vi "Tosca-Set Next Adapt Trial.vi"(0 "Track in":T4, 5 "change":bool, 7 "Track":T1, 9 "catch is tracked":bool) -> (4 "Track out":T4)   [LabVIEW 2020]
uses:
  Typedefs/Tosca-Adaptation Track State.ctl
  Typedefs/Tosca-Adaptation History Element.ctl
  Typedefs/Tosca-Adaptive Track.ctl
  Typedefs/Tosca-Simple Variable.ctl
  Tosca-Adapt Threshold Metric.ctl
  epl-vi-lib/Utility VIs/Array Manipulation VIs/Array-Dimensions (2D).vi
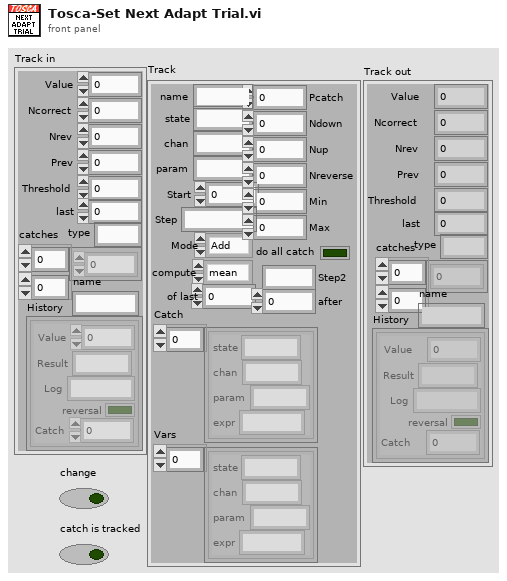
[diagram p1: front panel]
types:
  T1 = typedef "Tosca-Adaptive Track.ctl" = cluster{"state":string, "chan":string, "param":string, "Start":dbl, "Step":string, "Mode":enum16{"Add", "Multiply"}, "Pcatch":dbl, "Ndown":i32, "Nup":i32, "Nreverse":i32, "Min":dbl, "Max":dbl, "Catch":T2[], "do all catch":bool, "name":string, "Vars":T2[], "compute":T3, "of last":i32, "Step2":string, "after":i32}
  T2 = typedef "Tosca-Simple Variable.ctl" = cluster{"state":string, "chan":string, "param":string, "expr":string}
  T3 = typedef "Tosca-Adapt Threshold Metric.ctl" = enum16{"mean", "median"}
  T4 = typedef "Tosca-Adaptation Track State.ctl" = cluster{"Value":dbl, "Ncorrect":i32, "Nrev":i32, "Prev":dbl, "History":T5[], "Threshold":dbl, "last":i32, "type":string, "catches":dbl[][], "name":string}
  T5 = typedef "Tosca-Adaptation History Element.ctl" = cluster{"Value":dbl, "Result":string, "Log":string, "reversal":bool, "Catch":dbl}
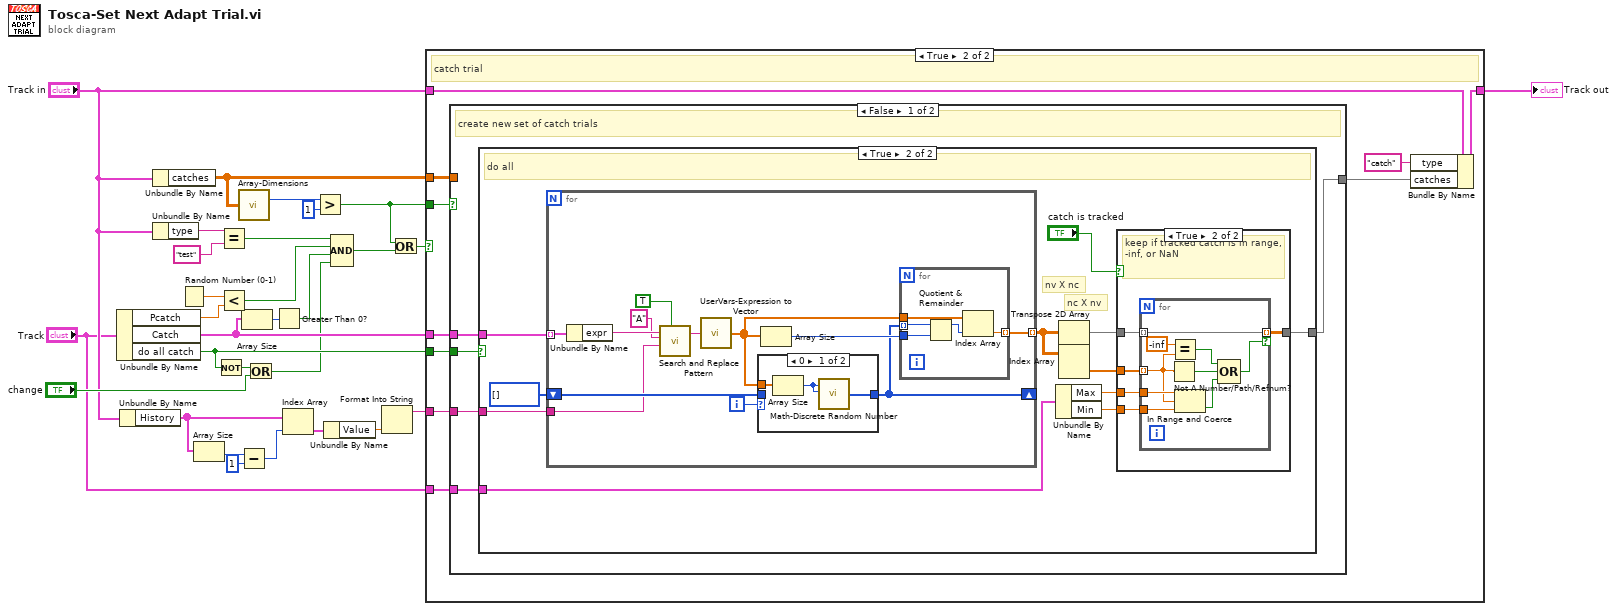
[diagram p0: block diagram]
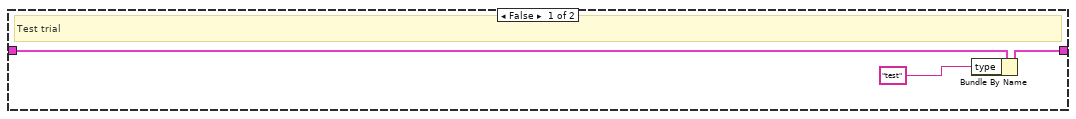
[diagram p2: hidden frame]
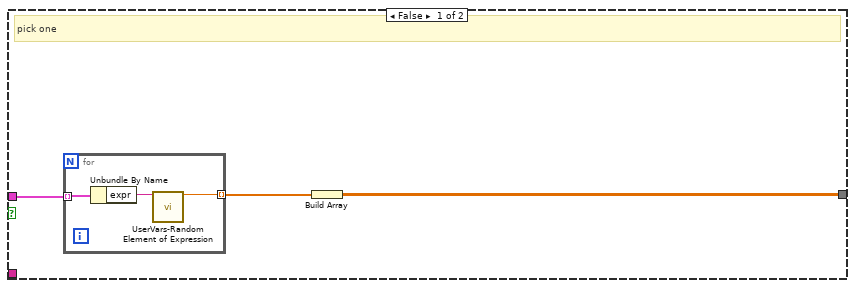
[diagram p3: hidden frame]
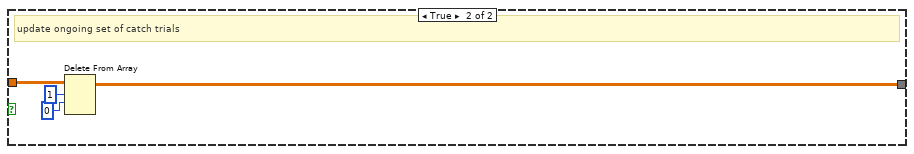
[diagram p6: hidden frame]
diagram:
  n1 = Unbundle By Name("Track") -> ("Pcatch"=w17:dbl, "Catch"=w16:T2[], "do all catch"=w13:bool)
  n2 = Unbundle By Name("Track in") -> ("History"=w4:T5[])
  n3 = Unbundle By Name("Track in") -> ("catches"=w21:dbl[][])
  n4 = Unbundle By Name("Track in") -> ("type"=w22:string)
  n5 = Random Number (0-1)() -> (number: 0 to 1=w24:dbl)
  n6 = Array Size(array=w4) -> (size(s)=w7:i32)
  n7 = Not(x=w13) -> (.not. x?=w12:bool)
  n8 = Equal?(x=w22, y="test") -> (x = y?=w25:bool)
  n9 = Less?(x=w24, y=w17) -> (x < y?=w26:bool)
  n10 = call-poly "Array-Dimensions.vi"("2D Array"=w21) -> ("# rows"=w19:i32)  [unwired: 13 in, 1 out]
  n11 = Subtract(x=w7, y=1) -> (x-y=w5:i32)
  n12 = Array Size(array=w16) -> (size(s)=w15:i32)
  n13 = Or(x=w12, y="change") -> (x .or. y?=w10:bool)
  n14 = Greater Than 0?(x=w15) -> (x > 0?=w14:bool)
  n15 = Index Array(array=w4, index=w5) -> (element=w3:T5)
  n16 = Greater?(x=w19, y=1) -> (0:w20:bool)
  n17 = Unbundle By Name(w3) -> ("Value"=w2:dbl)
  n18 = Compound Arithmetic op=AND(w25, w26, w14, w10) -> (w27:bool)
  n19 = Format Into String(w2) -> (resulting string=w8:string)  [unwired: 3 in, 1 out]
  n20 = Or(x=w20, y=w27) -> (x .or. y?=w28:bool)
  n21 = case shown="True" w28 {
    tunnel: "Track in" -> [w32 w42]
    tunnel: [w31 w39] -> w29
    tunnel: w21 -> [_ w40]
    tunnel: w20 -> [_ w41]
    tunnel: w16 -> [_ w36]
    tunnel: w13 -> [_ w35]
    tunnel: w8 -> [_ w34]
    tunnel: "Track" -> [_ w33]
    frame False {
      # "Test trial"
      n22 = Bundle By Name(cluster=w32, "type"="test") -> (w31:T4)
    }
    frame True {
      # "catch trial"
      n23 = case shown="False" w41 {
        tunnel: w40 -> [_ w104]
        tunnel: [w45 w102] -> w38
        tunnel: w36 -> [w46 _]
        tunnel: w35 -> [w47 _]
        tunnel: w34 -> [w44 _]
        tunnel: w33 -> [w43 _]
        frame False {
          # "create new set of catch trials"
          n24 = case shown="True" w47 {
            tunnel: w46 -> [w50 w64]
            tunnel: [w48 w56] -> w45
            tunnel: w44 -> [_ w63]
            tunnel: w43 -> [_ w62]
            frame False {
              # "pick one"
              n25 = for {
                tunnel: w50 -> [w53] mode=indexing
                tunnel: [w51] -> w49 mode=indexing
                n26 = Unbundle By Name(w53) -> ("expr"=w52:string)
                n27 = call "UserVars-Random Element of Expression.vi"("Expr"=w52) -> ("Random Element"=w51:dbl)  [unwired: 12 in, 2 out]
              }
              n28 = Build Array(w49) -> (w48:dbl[][])
            }
            frame True {
              # "nc X nv"
              # "nv X nc"
              # "do all"
              n29 = for {
                tunnel: w64 -> [w91] mode=indexing
                shift-right: [w80] -> _
                shift-left: i32[] [] -> [w90]
                tunnel: [w87] -> w61 mode=indexing
                tunnel: w63 -> [w83]
                i -> [w89]
                n30 = Unbundle By Name(w91) -> ("expr"=w85:string)
                n31 = call <vilib>:"Search and Replace Pattern.vi"("string"=w85, "regular expression (\"\")"="A" ("regular expression (\"\")"), "replace string (\"\")"=w83, "replace all? (F)"=TRUE) -> ("result string"=w86:string)  [unwired: 1 in, 1 out]
                n32 = call "UserVars-Expression to Vector.vi"("Expr"=w86) -> ("Values"=w88:dbl[])  [unwired: 13 in, 1 out]
                n33 = case shown="0" w89 {
                  tunnel: w88 -> [w99 _]
                  tunnel: w90 -> [_ w100]
                  tunnel: [w97 w100] -> w80
                  frame 0 {
                    n34 = Array Size(array=w99) -> (size(s)=w98:i32)
                    n35 = call "Math-Discrete Random Number.vi"("N"=w98, "samples"=w98) -> ("Random Values"=w97:i32[])  [unwired: 4 in]
                  }
                  frame 1, Default {
                  }
                }
                n36 = Array Size(array=w88) -> (size(s)=w81:i32)
                n37 = for {
                  tunnel: w88 -> [w96]
                  tunnel: [w95] -> w87 mode=indexing
                  tunnel: w81 -> [w93]
                  tunnel: w80 -> [w92] mode=indexing
                  n38 = Quotient & Remainder(x=w92, y=w93) -> (x-y*floor(x/y)=w94:i32)  [unwired: 1 out]
                  n39 = Index Array(array=w96, index=w94) -> (element=w95:dbl)
                }
              }
              n40 = Unbundle By Name(w62) -> ("Max"=w59:dbl, "Min"=w58:dbl)
              n41 = Transpose 2D Array(2D array=w61) -> (transposed array=w57:dbl[][])
              n42 = Index Array(array=w61) -> (element=w60:dbl[])  [unwired: 2 in]
              n43 = case shown="True" "catch is tracked" {
                tunnel: w60 -> [_ w70]
                tunnel: w59 -> [_ w69]
                tunnel: w58 -> [_ w68]
                tunnel: w57 -> [w65 w67]
                tunnel: [w65 w66] -> w56
                frame False {
                }
                frame True {
                  # "keep if tracked catch is in range, -inf, or NaN"
                  n44 = for {
                    tunnel: w67 -> [w77] mode=indexing
                    tunnel: w70 -> [w72] mode=indexing
                    tunnel: w69 -> [w79]
                    tunnel: w68 -> [w78]
                    tunnel: [w77] -> w66 mode=indexing if=w74
                    n45 = Not A Number/Path/Refnum?(number/path/refnum=w72) -> (NaN/Path/Refnum?=w76:bool)
                    n46 = Equal?(x=-inf, y=w72) -> (x = y?=w73:bool)
                    n47 = In Range and Coerce(upper limit=w79, x=w72, lower limit=w78) -> (In Range?=w75:bool)  [unwired: 1 out]
                    n48 = Compound Arithmetic op=OR(w73, w76, w75) -> (w74:bool)
                  }
                }
              }
            }
          }
        }
        frame True {
          # "update ongoing set of catch trials"
          n49 = Delete From Array(array=w104, length=1, index (row)=0) -> (array with subset deleted=w102:dbl[][])  [unwired: 1 in, 1 out]
        }
      }
      n50 = Bundle By Name(cluster=w42, "type"="catch", "catches"=w38) -> (w39:T4)
    }
  }
  "Track out" <- w29
